vi "Data base.vi"() -> ()   [LabVIEW 2017]
uses:
  Control 1.ctl
panel:
  in  "Search Field":T1
  in  "stop":bool
  in  "Validity":dbl
  out "Details 3":T2
  in  "Card Number":dbl
  out "Details 2":T2
  out "Details":T2
  in  "Card Holder":string
  in  "Account Details":T3(array[cluster])
  # "DataBase"
  # "Search Box"
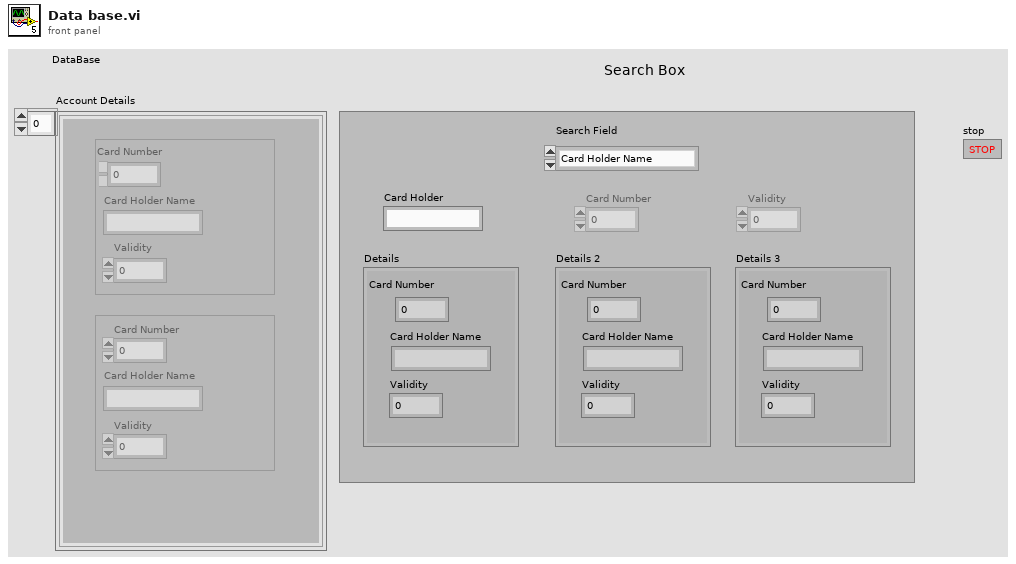
[diagram p1: front panel]
types:
  T1 = typedef "Control 1.ctl" = enum16{"Card Holder Name", "Card Number", "Validity"}
  T2 = cluster{" Card Number":dbl, "Card Holder Name":string, "Validity":dbl}
  T3 = cluster{cluster{"Numeric":dbl, "Card Holder Name":string, "Validity":dbl}, cluster{"Numeric":dbl, "Card Holder Name":string, "Validity":dbl}}[]
  T4 = enum8{"Enabled", "Disabled", "Disabled and Grayed Out"}
  T5 = cluster{cluster{"Numeric":dbl, "Card Holder Name":string, "Validity":dbl}, cluster{"Numeric":dbl, "Card Holder Name":string, "Validity":dbl}}
  T6 = cluster{"Numeric":dbl, "Card Holder Name":string, "Validity":dbl}
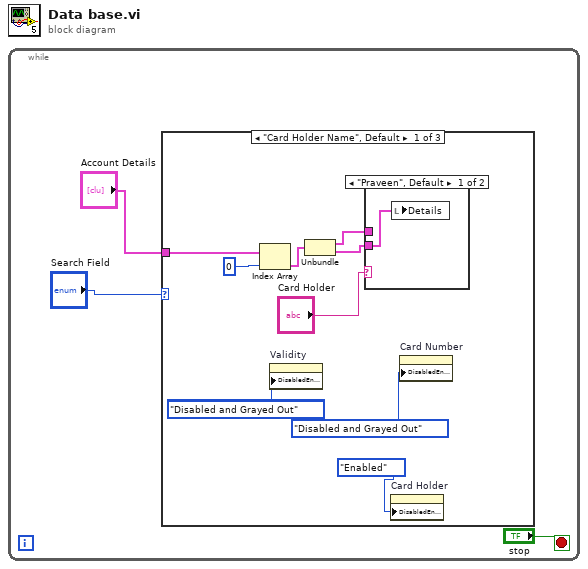
[diagram p0: block diagram]
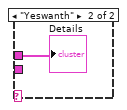
[diagram p2: hidden frame]
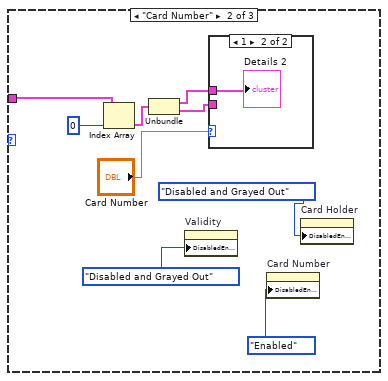
[diagram p3: hidden frame]
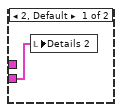
[diagram p4: hidden frame]
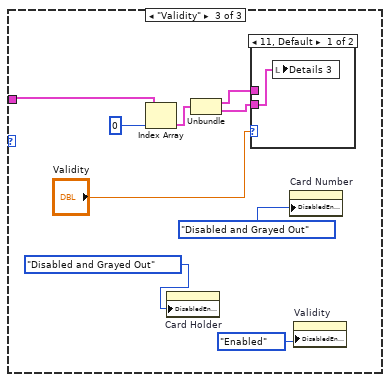
[diagram p5: hidden frame]
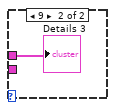
[diagram p6: hidden frame]
diagram:
  n1 = while {
    stop <- "stop" stop-if-true
    n2 = case shown="\"Card Holder Name\", Default" "Search Field" {
      tunnel: "Account Details" -> [w7 w19 w30]
      frame "Card Holder Name", Default {
        (unwired) T4."Disabled and Grayed Out" ("Disabled 2")
        n3 = Index Array(array=w7, index=0) -> (element=w11:T5)
        n4 = property on="Validity" class="DigNum (strict)"("DisabledEnum"=T4."Disabled and Grayed Out" ("Disabled 2")) -> ()  [unwired: 2 in, 2 out]
        n5 = Unbundle(w11) -> (w10:T6, w9:T6)
        n6 = case shown="\"Praveen\", Default" "Card Holder" {
          tunnel: w10 -> [_ w14]
          tunnel: w9 -> [w13 _]
          frame "Praveen", Default {
            n7 = local write "Details"(w13) -> ()
          }
          frame "Yeswanth" {
            "Details" <- w14
          }
        }
        n8 = property on="Card Holder" class="Str"("DisabledEnum"=T4."Enabled" ("Disabled 3")) -> ()  [unwired: 2 in, 2 out]
        n9 = property on="Card Number" class="DigNum (strict)"("DisabledEnum"=T4."Disabled and Grayed Out" ("Disabled")) -> ()  [unwired: 2 in, 2 out]
      }
      frame "Card Number" {
        n10 = Index Array(array=w19, index=0) -> (element=w23:T5)
        n11 = Unbundle(w23) -> (w22:T6, w21:T6)
        n12 = property on="Validity" class="DigNum (strict)"("DisabledEnum"=T4."Disabled and Grayed Out" ("Disabled 2")) -> ()  [unwired: 2 in, 2 out]
        n13 = case shown="1" "Card Number" {
          tunnel: w22 -> [_ w25]
          tunnel: w21 -> [w24 _]
          frame 2, Default {
            n14 = local write "Details 2"(w24) -> ()
          }
          frame 1 {
            "Details 2" <- w25
          }
        }
        n15 = property on="Card Number" class="DigNum (strict)"("DisabledEnum"=T4."Enabled" ("Disabled")) -> ()  [unwired: 2 in, 2 out]
        n16 = property on="Card Holder" class="Str"("DisabledEnum"=T4."Disabled and Grayed Out" ("Disabled 3")) -> ()  [unwired: 2 in, 2 out]
      }
      frame "Validity" {
        n17 = Index Array(array=w30, index=0) -> (element=w34:T5)
        n18 = property on="Card Holder" class="Str"("DisabledEnum"=T4."Disabled and Grayed Out" ("Disabled 3")) -> ()  [unwired: 2 in, 2 out]
        n19 = Unbundle(w34) -> (w33:T6, w32:T6)
        n20 = case shown="11, Default" "Validity" {
          tunnel: w33 -> [_ w36]
          tunnel: w32 -> [w35 _]
          frame 11, Default {
            n21 = local write "Details 3"(w35) -> ()
          }
          frame 9 {
            "Details 3" <- w36
          }
        }
        n22 = property on="Card Number" class="DigNum (strict)"("DisabledEnum"=T4."Disabled and Grayed Out" ("Disabled")) -> ()  [unwired: 2 in, 2 out]
        n23 = property on="Validity" class="DigNum (strict)"("DisabledEnum"=T4."Enabled" ("Disabled")) -> ()  [unwired: 2 in, 2 out]
      }
    }
  }
